vi "Self-Test.vi"(8 "error in (no error)":errorcluster, 11 "MSOX6004 in":refnum<class "MSOX6004.lvclass">) -> (0 "error out":errorcluster, 2 "Self-Test Passed? (T:Yes)":bool, 3 "MSOX6004 out":refnum<class "MSOX6004.lvclass">)   [LabVIEW 2018, in "MSOX6004.lvlib" / "MSOX6004.lvclass"]
doc: "This Override method is used to call the Self-Test function of the Oscope instrument. The boolean output 'Self-Test Passed? (T:Yes)' carries out the Self-Test result."
uses:
  MSOX6004.lvclass
  MSOX6004.lvclass/MSOX6004.ctl
  <instrlib>/Keysight InfiniiVision/Keysight InfiniiVision.lvlib
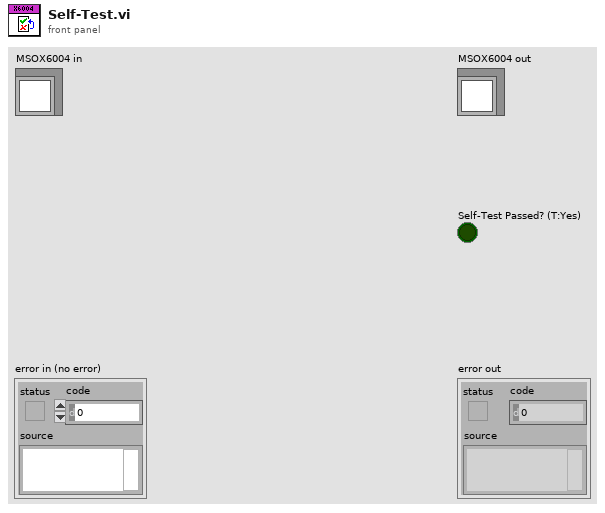
[diagram p1: front panel]
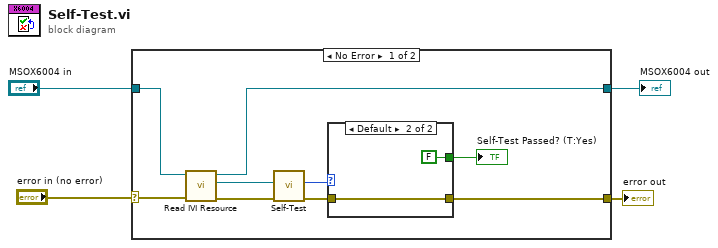
[diagram p0: block diagram]
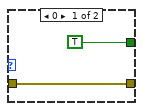
[diagram p2: hidden frame]
diagram:
  n1 = case shown="No Error" "error in (no error)" {
    selector: "error in (no error)" -> [w13 w18]
    tunnel: [w10 w19] -> w3
    tunnel: "MSOX6004 in" -> [w12 w19]
    tunnel: [w6 w18] -> w1
    frame No Error {
      n2 = call "Read IVI Resource.vi"("error in (no error)"=w13, "MSOX6004 in"=w12) -> ("error out"=w11:errorcluster, "IVI Resource"=w9:refnum<k15>, "MSOX6004 out"=w10:refnum<class "MSOX6004.lvclass">)  [unwired: 7 in]
      n3 = call <instrlib>:"Self-Test.vi"("error in (no error)"=w11, "instrument handle"=w9) -> ("error out"=w5:errorcluster, "self test result"=w8:i16)  [unwired: 6 in, 2 out]
      n4 = case shown="Default" w8 {
        tunnel: [TRUE FALSE] -> w7
        tunnel: [w14 w16] -> w6
        tunnel: w5 -> [w14 w16]
        frame 0 {
        }
        frame Default {
        }
      }
      "Self-Test Passed? (T:Yes)" <- w7
    }
    frame Error {
    }
  }
  "error out" <- w1
  "MSOX6004 out" <- w3
